vi "启动整机测试 (子VI).vi"() -> (0 "error out":T1={"status"=FALSE, "代码"=4, "source"=""} caption="错误输出" {"代码" items=["执行成功"=1, "执行失败，但不知道原因"=2, "命令请求条件错误"=3, "通讯超时"=4, "系统繁忙不能执行"=5, "系统故障"=6, "没有数据"=100]})   [LabVIEW 2016]
uses:
  PLC/PLC.lvlib
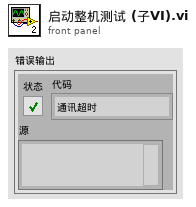
[diagram p1: front panel]
types:
  T1 = cluster{"status":bool, "代码":u16, "source":string}
  T2 = enum32{"Bad", "Idle", "Run top level", "Running"}
  T3 = cluster{"氨氮":bool, "总磷":bool, "总氮":bool, "多参数":bool, "CODMn":bool, "CODcr":bool}
  T4 = cluster{"测试模式":enum16{"正常测试", "集成干预"}, "参数启用":cluster{"氨氮":bool, "总磷":bool, "总氮":bool, "多参数":bool, "CODMn":bool, "CODcr":bool}}
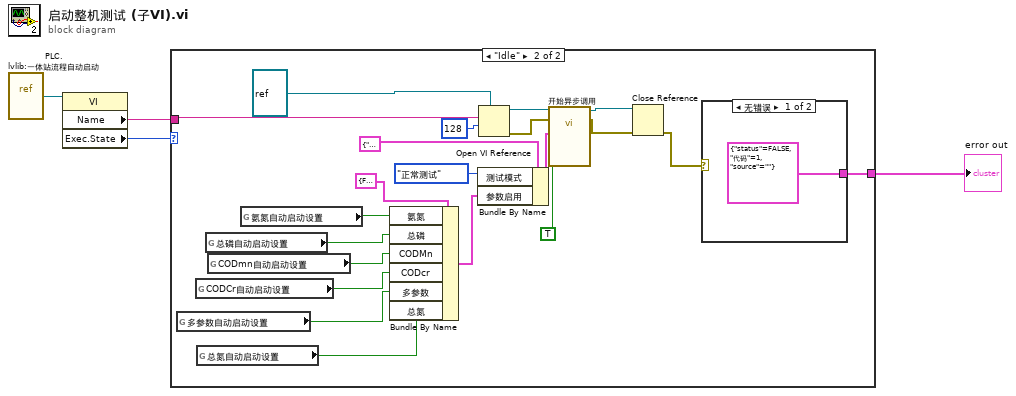
[diagram p0: block diagram]
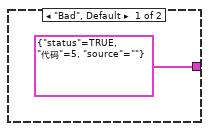
[diagram p2: hidden frame]
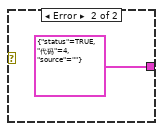
[diagram p3: hidden frame]
diagram:
  n1 = vi-ref "PLC.lvlib:一体站流程自动启动.vi"() -> (w3:refnum<vi>)
  n2 = property class="VI"(reference=w3) -> ("Name"=w4:string, "Exec.State"=w2:T2)  [unwired: 1 in, 2 out]
  n3 = case shown="\"Idle\"" w2 {
    tunnel: w4 -> [_ w21]
    tunnel: [T1 {"status"=TRUE, "代码"=5, "source"=""} ("error out") w19] -> w1
    frame "Bad", Default {
    }
    frame "Idle" {
      n4 = global read "系统设置全局变量.vi" "多参数自动启动设置"() -> (w12:bool)
      n5 = global read "系统设置全局变量.vi" "CODCr自动启动设置"() -> (w13:bool)
      n6 = global read "系统设置全局变量.vi" "总氮自动启动设置"() -> (w9:bool)
      n7 = global read "系统设置全局变量.vi" "总磷自动启动设置"() -> (w15:bool)
      n8 = global read "系统设置全局变量.vi" "CODmn自动启动设置"() -> (w14:bool)
      n9 = global read "系统设置全局变量.vi" "氨氮自动启动设置"() -> (w16:bool)
      n10 = Bundle By Name(cluster=T3 {"氨氮"=FALSE, "总磷"=FALSE, "总氮"=FALSE, "多参数"=FALSE, "CODMn"=FALSE, "CODcr"=FALSE} ("参数启用"), "氨氮"=w16, "总磷"=w15, "CODMn"=w14, "CODcr"=w13, "多参数"=w12, "总氮"=w9) -> (w8:T3)
      n11 = Bundle By Name(cluster=T4 {"测试模式"=enum."正常测试", "参数启用"={"氨氮"=FALSE, "总磷"=FALSE, "总氮"=FALSE, "多参数"=FALSE, "CODMn"=FALSE, "CODcr"=FALSE}} ("参数"), "测试模式"=enum16{"正常测试", "集成干预", "加标回收"}."正常测试", "参数启用"=w8) -> (w7:T4)
      n12 = Open VI Reference(type specifier VI Refnum (for type only)=refnum<vi> refnum, vi path=w21, options=128 ("选项")) -> (vi reference=w23:refnum<vi>, error out=w25:errorcluster)  [unwired: 3 in]
      n13 = call-by-ref "开始异步调用"(reference=w23, error in=w25, "二级进样"=TRUE, "参数"=w7) -> (reference out=w24:refnum<vi>, error out=w26:errorcluster)  [unwired: 10 in]
      n14 = Close Reference(reference=w24, error in (no error)=w26) -> (error out=w18:errorcluster)
      n15 = case shown="无错误" w18 {
        tunnel: [T1 {"status"=FALSE, "代码"=1, "source"=""} ("error out") T1 {"status"=TRUE, "代码"=4, "source"=""} ("error out")] -> w19
        frame No Error {
        }
        frame Error {
        }
      }
    }
  }
  "error out" <- w1
